vi "JFW_ATTEN.vi"() -> ()   [LabVIEW 2020]
uses:
  <vilib>/Instr/_visa.llb/VISA Configure Serial Port (Instr).vi
panel:
  in  "String":string
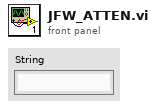
[diagram p1: front panel]
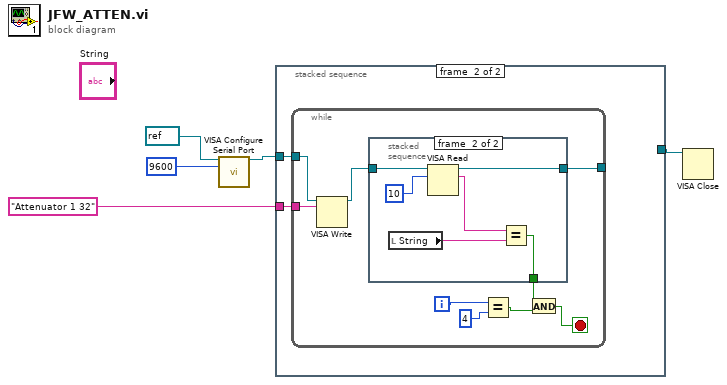
[diagram p0: block diagram]
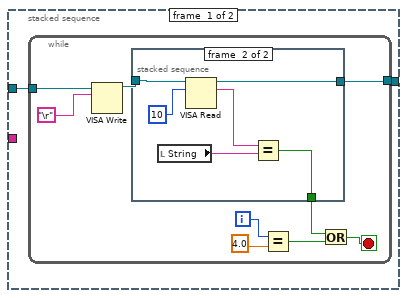
[diagram p2: hidden frame]
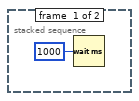
[diagram p3: hidden frame]
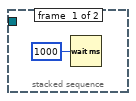
[diagram p4: hidden frame]
diagram:
  n1 = call-poly "VISA Configure Serial Port"("VISA resource name"=refnum<visa-resource-name> refnum, "baud rate (9600)"=u32 9600) -> ("VISA resource name out"=w3:refnum<visa-resource-name>)  [unwired: 12 in, 1 out]
  n2 = stacked-sequence {
    tunnel: w3 -> [w7 w24]
    tunnel: "Attenuator 1 32" ("write buffer") -> [_ w25]
    tunnel: [w6 _] -> w1
    frame #0 {
      n3 = while {
        tunnel: w7 -> [w15]
        tunnel: [w11] -> w6
        i -> [w14]
        stop <- w8 stop-if-true
        n4 = VISA Write(VISA resource name=w15, write buffer="\r") -> (VISA resource name out=w10:refnum<visa-resource-name>)  [unwired: 1 in, 2 out]
        n5 = stacked-sequence {
          tunnel: w10 -> [_ w20]
          tunnel: [_ w22] -> w11
          tunnel: [_ w21] -> w9
          frame #0 {
            n6 = Wait (ms)(milliseconds to wait=u32 1000) -> ()  [unwired: 1 out]
          }
          frame #1 {
            n7 = local read "String"() -> (w18:string)
            n8 = VISA Read(VISA resource name=w20, byte count=u32 10) -> (VISA resource name out=w22:refnum<visa-resource-name>, read buffer=w23:string)  [unwired: 1 in, 2 out]
            n9 = Equal?(x=w23, y=w18) -> (x = y?=w21:bool)
          }
        }
        n10 = Equal?(x=w14, y=4.0) -> (x = y?=w12:bool)
        n11 = Or(x=w9, y=w12) -> (x .or. y?=w8:bool)
      }
    }
    frame #1 {
      n12 = while {
        tunnel: w25 -> [w34]
        tunnel: w24 -> [w33]
        tunnel: [w30] -> _
        i -> [w32]
        stop <- w28 stop-if-true
        n13 = VISA Write(VISA resource name=w33, write buffer=w34) -> (VISA resource name out=w29:refnum<visa-resource-name>)  [unwired: 1 in, 2 out]
        n14 = stacked-sequence {
          tunnel: [_ w40] -> w27
          tunnel: w29 -> [_ w38]
          tunnel: [_ w39] -> w30
          frame #0 {
            n15 = Wait (ms)(milliseconds to wait=u32 1000) -> ()  [unwired: 1 out]
          }
          frame #1 {
            n16 = local read "String"() -> (w36:string)
            n17 = VISA Read(VISA resource name=w38, byte count=u32 10) -> (VISA resource name out=w39:refnum<visa-resource-name>, read buffer=w41:string)  [unwired: 1 in, 2 out]
            n18 = Equal?(x=w41, y=w36) -> (x = y?=w40:bool)
          }
        }
        n19 = Equal?(x=w32, y=4) -> (x = y?=w26:bool)
        n20 = And(x=w27, y=w26) -> (x .and. y?=w28:bool)
      }
    }
  }
  n21 = VISA Close(VISA resource name=w1) -> ()  [unwired: 1 in, 1 out]
